vi "Power Measure Call Back.vi"(5 "iTriggerLevel":i32, 6 "iTriggerType":u32, 7 "iNumAvg":u32, 8 "error in (no error)":errorcluster, 9 "dPowerLevel":dbl, 10 "iFreq":u32, 11 "iGain":u32) -> (0 "error out":errorcluster, 3 "function return":dbl)   [LabVIEW 2013, in "QCAWLAN_DLL.lvlib"]
doc: "QCA_DLL_Export double PowerMeasureCallBack(unsigned int iGain, unsigned int iFreq, double dPowerLevel, unsigned int iNumAvg, unsigned int iTriggerType, int iTriggerLevel);"
uses:
  QCAWLAN_DLL.lvlib
  QCAWLAN_DLL.dll
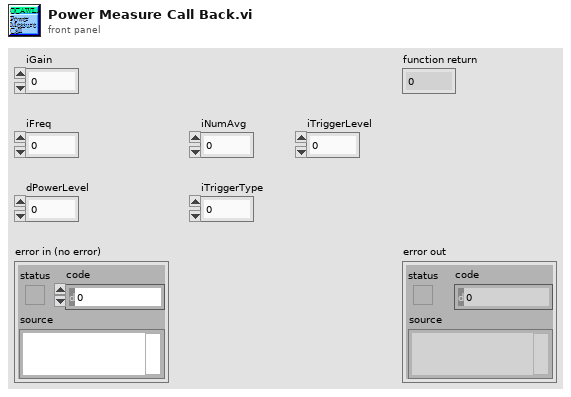
[diagram p1: front panel]
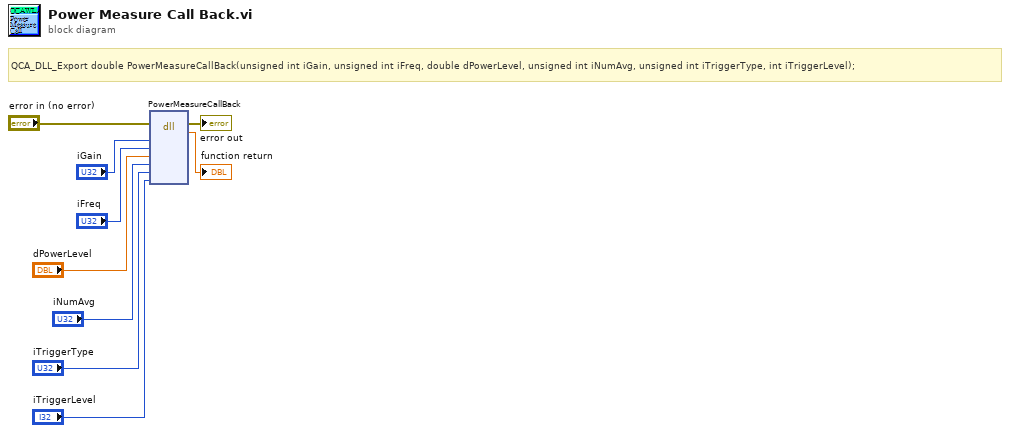
[diagram p0: block diagram]
diagram:
  # "QCA_DLL_Export double PowerMeasureCallBack(unsigned int iGain, unsigned int iFreq, double dPowerLevel, unsigned int iNumAvg, unsigned int iTriggerType, int iTriggerLevel);"
  n1 = dll-call lib="C:/Users/dave_yao/Desktop/Hitron/QCA9984 WLAN_LV2013/user.lib/QCAWLAN_DLL/QCAWLAN_DLL.*" fn="PowerMeasureCallBack"(error in="error in (no error)", "iGain"="iGain", "iFreq"="iFreq", "dPowerLevel"="dPowerLevel", "iNumAvg"="iNumAvg", "iTriggerType"="iTriggerType", "iTriggerLevel"="iTriggerLevel") -> (error out=→"error out":errorcluster, →"function return":dbl)  [unwired: 8 in, 1 out]
